vi "direk.vi"() -> ()   [LabVIEW 2019]
uses:
  <vilib>/sound2/lvsound2.llb/Sound File Refnum.ctl
  <vilib>/sound2/lvsound2.llb/Sound Data Format.ctl
  <vilib>/Analysis/baseanly.llb/Mean (DBL).vi
  <vilib>/Waveform/WDTOps.llb/WDT Waveform to XY Pairs DBL.vi
  <vilib>/express/express analysis/Spectral/Block/exnSpectralBlock spectral measurements RMS poly.vi
  <vilib>/express/express analysis/Spectral/Block/exnSpectralBlock spectral measurements RMS WFM.vi
  <vilib>/sound2/lvsound2.llb/Sound File Write Open.vi
  <vilib>/sound2/lvsound2.llb/Sound File Write (DBL Single).vi
  <vilib>/express/express analysis/Spectral/XNode/ExpressSpectralMeasurementsBlockNode.xnode
  <vilib>/Analysis/NI_AALBase.lvlib
  newdll/Dll12/x64/Debug/Dll12.dll
panel:
  out "Noise Std":dbl[](graph) caption="Data"
  out "noise type":string
  out "mean":dbl format="%0.2f"
  out "Noise type":dbl[](graph) caption="Data"
  out "Energy":dbl[](graph) caption="Data"
  in  "sound format":T1={"sample rate (S/s)"=22050.0, "number of channels"=2, "bits per sample"=16}
  in  "path 2":path
  out "sound file refnum":T2
  in  "Do you want to save?":bool
  in  "P":u64
  out "FFT OF CLEAN":cluster{"f0":dbl, "df":dbl, "magnitude":dbl[]}(graph) caption="Data"
  out "FFT OF INPUT":cluster{"f0":dbl, "df":dbl, "magnitude":dbl[]}(graph) caption="Data"
  out "Clean Time":waveform(dbl)(graph)
  in  "stop":bool
  in  "Device 2":u32 caption="Device"
  out "size(s)":i32
  out "Input":waveform(dbl)(graph)
  in  "path":path
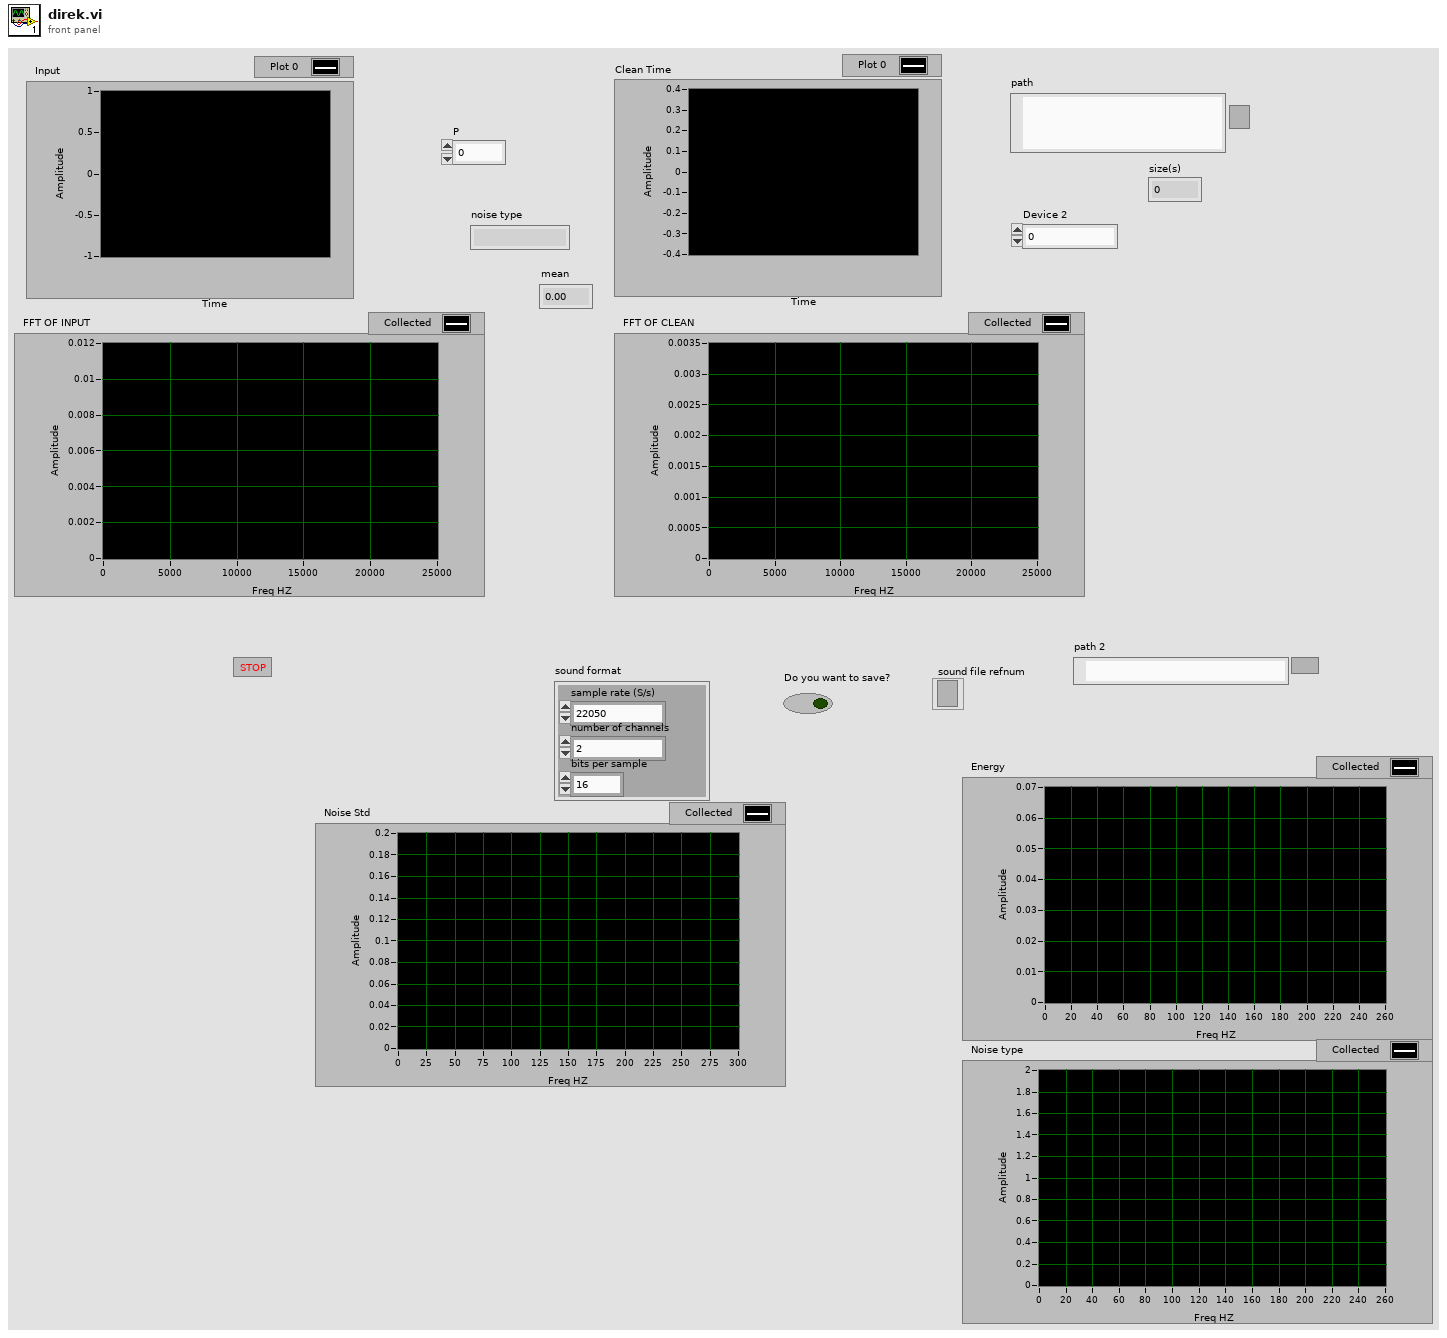
[diagram p1: front panel]
types:
  T1 = typedef "Sound Data Format.ctl" = cluster{"sample rate (S/s)":dbl, "number of channels":i32, "bits per sample":i32}
  T2 = typedef "Sound File Refnum.ctl" = refnum<file>
  T3 = cluster{"averaging mode":u16, "weighting mode":u16, "number of averages":u32}
  T4 = cluster{"dB On (F)":bool, "unwrap phase (F)":bool, "convert to degree (F)":bool}
  T5 = cluster{"data[0]":waveform(dbl), "data[1]":waveform(dbl), "data[2]":waveform(dbl), "data[3]":waveform(dbl), "data[4]":waveform(dbl), "data[5]":waveform(dbl), "data[6]":waveform(dbl), "data[7]":waveform(dbl), "data[8]":waveform(dbl)}
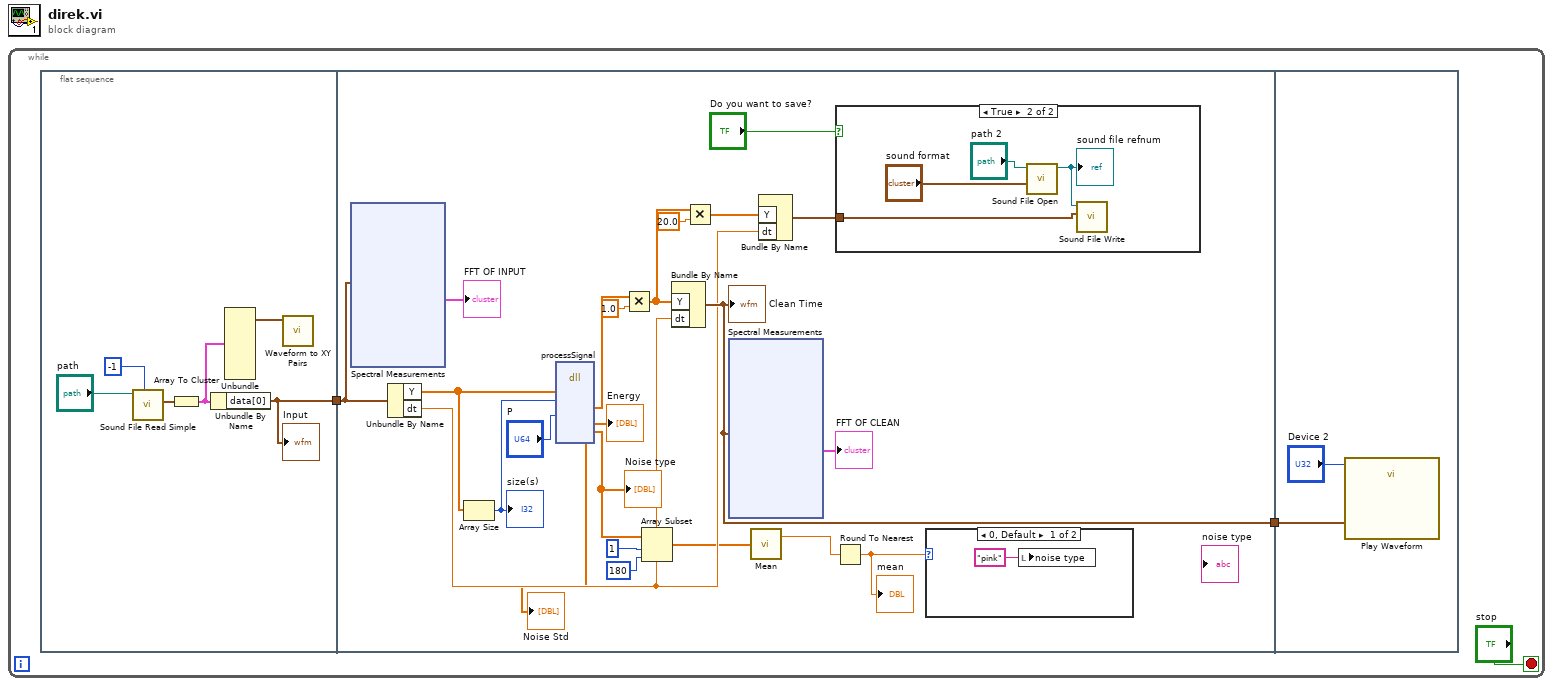
[diagram p0: block diagram]
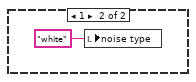
[diagram p2: hidden frame]
diagram:
  n1 = while {
    stop <- "stop" stop-if-true
    n2 = flat-sequence {
      tunnel: [w7] -> w2
      tunnel: w2 -> [w29]
      tunnel: [w25] -> w1
      tunnel: w1 -> [w59]
      frame #0 {
        n3 = call <vilib>:"Sound File Read Simple.vi"("number of samples/ch (-1: all)"=-1, "path"="path") -> ("data"=w4:waveform(dbl)[])  [unwired: 6 in, 3 out]
        n4 = Array To Cluster(array=w4) -> (cluster=w8:T5)
        n5 = Unbundle By Name(w8) -> ("data[0]"=w7:waveform(dbl))
        "Input" <- w7
        n6 = Unbundle(w8) -> ("data[1]"=w9:waveform(dbl))  [unwired: 8 out]
        n7 = call-poly <vilib>:"Waveform to XY Pairs.vi"("waveform in"=w9) -> ()  [unwired: 8 in, 3 out]
      }
      frame #1 {
        n8 = xnode "Spectral Measurements"("Signals"=w29) -> ("FFT - (RMS)"=→"FFT OF INPUT":cluster{"f0":dbl, "df":dbl, "magnitude":dbl[]})  [unwired: 1 in, 2 out]
        n9 = Unbundle By Name(w29) -> ("Y"=w19:dbl[], "dt"=w21:dbl)
        n10 = Array Size(array=w19) -> (size(s)=w18:i32)
        "size(s)" <- w18
        n11 = dll-call lib="C:/Users/Yunus/Desktop/newdll/Dll12/x64/Debug/Dll12.dll" fn="processSignal"("noisySignal"=w19, "signalLength"=w18, "P"="P") -> ("filteredSignal"=w31:dbl[], "speecher"=→"Energy":dbl[], "noisetype"=w13:dbl[], "noisestd"=→"Noise Std":dbl[])  [unwired: 11 in, 2 out]
        "Noise type" <- w13
        n12 = Multiply(x=w31, y=1.0) -> (x*y=w22:dbl[])
        n13 = Array Subset(array=w13, index=1, length=180) -> (w12:dbl[])
        n14 = Bundle By Name("Y"=w22, "dt"=w21) -> (w25:waveform(dbl))  [unwired: 1 in]
        "Clean Time" <- w25
        n15 = Multiply(x=w22, y=20.0) -> (x*y=w23:dbl[])
        n16 = xnode "Spectral Measurements"("Signals"=w25) -> ("FFT - (RMS)"=→"FFT OF CLEAN":cluster{"f0":dbl, "df":dbl, "magnitude":dbl[]})  [unwired: 1 in, 2 out]
        n17 = call-poly <vilib>:"Mean.vi"("X"=w12) -> ("mean"=w16:dbl)  [unwired: 1 out]
        n18 = Bundle By Name("Y"=w23, "dt"=w21) -> (w20:waveform(dbl))  [unwired: 1 in]
        n19 = Round To Nearest(number=w16) -> (nearest integer value=w11:dbl)
        "mean" <- w11
        n20 = case shown="True" "Do you want to save?" {
          tunnel: w20 -> [_ w35]
          frame False {
          }
          frame True {
            n21 = call-poly <vilib>:"Sound File Open.vi"("sound format"="sound format", "path"="path 2") -> ("sound file refnum"=w38:T2)  [unwired: 8 in, 1 out]
            "sound file refnum" <- w38
            n22 = call-poly <vilib>:"Sound File Write.vi"("data"=w35, "sound file refnum"=w38) -> ()  [unwired: 8 in, 2 out]
          }
        }
        n23 = case shown="0, Default" w11 {
          frame 0, Default {
            n24 = local write "noise type"("pink" ("String 2")) -> ()
          }
          frame 1 {
            n25 = local write "noise type"("white" ("String")) -> ()
          }
        }
      }
      frame #2 {
        n26 = call "Play Waveform"("Device"="Device 2", "Data"=w59) -> ()  [unwired: 17 in, 1 out]
      }
    }
  }
